vi "CameraSetting_AdvanceAttributesDisplay.vi"(8 "error in (no error)":errorcluster caption="错误输入（无错误）", 11 "当前可用相机":string(combo)) -> (0 "error out":errorcluster caption="错误输出")   [LabVIEW 2015]
panel:
  in  "主页按钮":bool
  in  "刷新按钮":bool
  out "相机属性参数列表":string[][](table)
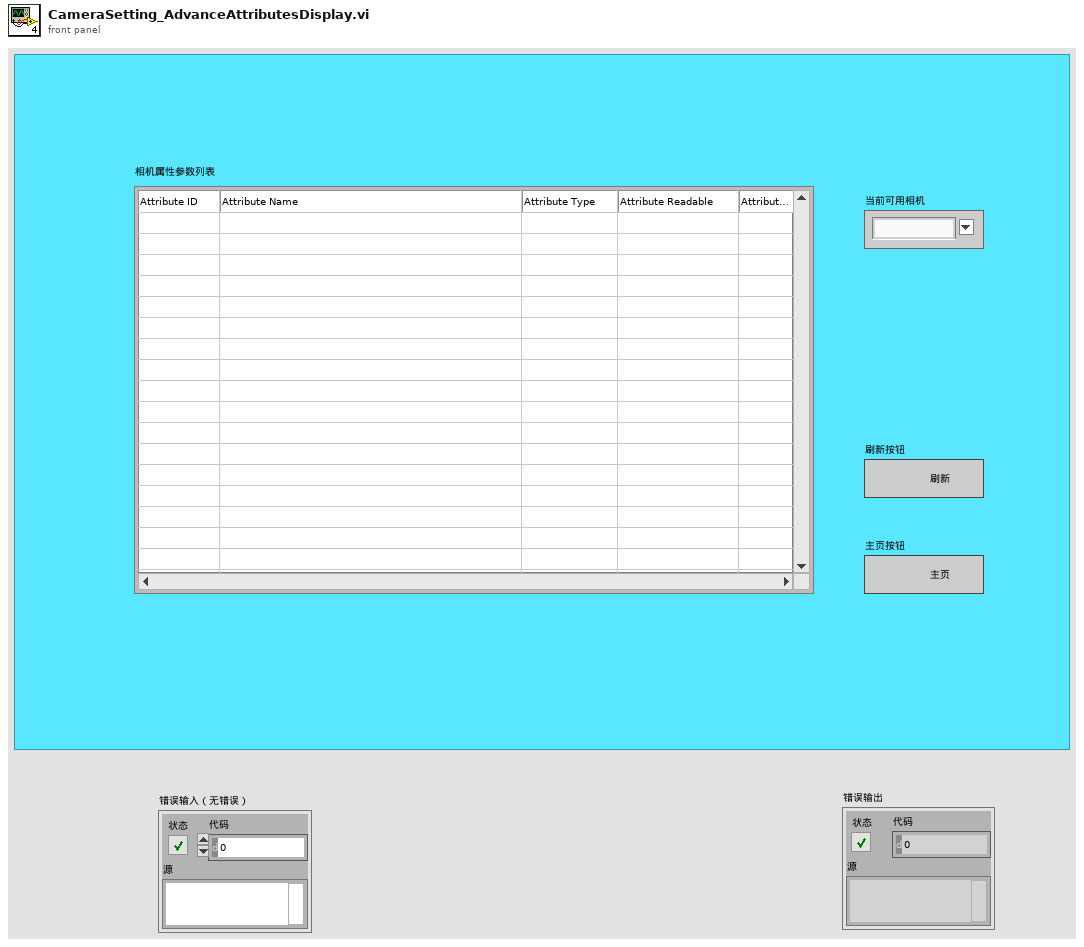
[diagram p1: front panel]
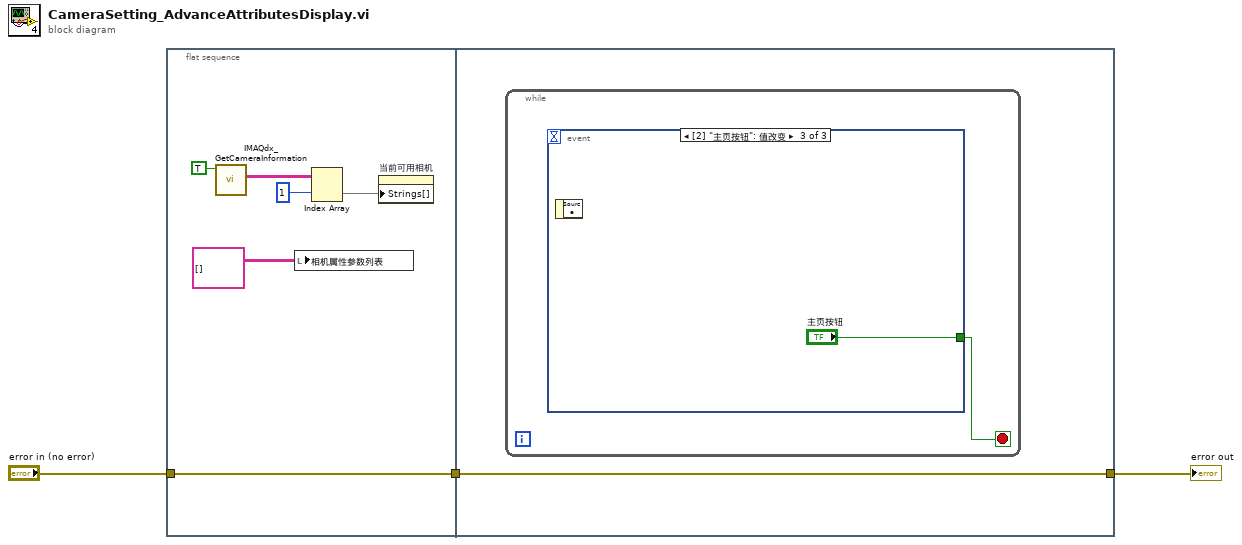
[diagram p0: block diagram]
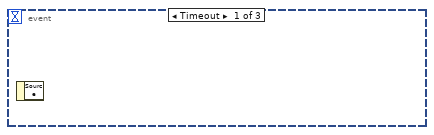
[diagram p2: hidden frame]
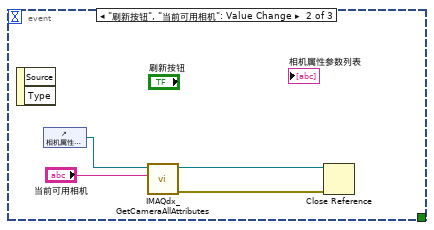
[diagram p3: hidden frame]
diagram:
  n1 = flat-sequence {
    tunnel: [w4] -> w3
    tunnel: "error in (no error)" -> [w4]
    tunnel: w3 -> [w10]
    tunnel: [w10] -> w1
    frame #0 {
      n2 = call "IMAQdx_GetCameraInformation.vi"("Connected Only? (Yes)"=TRUE) -> ("Camera Basic Information"=w9:string[][])  [unwired: 8 in, 2 out]
      n3 = local write "相机属性参数列表"(string[][] [] ("相机属性列表")) -> ()
      n4 = Index Array(array=w9, index (row)=1 ("索引 (行)")) -> (element=w7:string[])  [unwired: 1 in]
      n5 = property on="当前可用相机" class="CmbBox"("Strings[]"=w7) -> ()  [unwired: 2 in, 2 out]
    }
    frame #1 {
      n6 = while {
        stop <- w11 stop-if-true
        n7 = event shown="[2] \"主页按钮\": 值改变" {
          selector: _ -> [_ _ _]
          dyn-events: _ -> [_ _ _]
          timeout: _ -> [_ _ _]
          tunnel: [_ _ "主页按钮"] -> w11
          event Timeout {
            n8 = event-data() -> ()  [unwired: 1 in, 1 out]
          }
          event "刷新按钮", "当前可用相机": Value Change {
            n9 = event-data() -> ()  [unwired: 1 in, 2 out]
            n10 = control-ref of="相机属性参数列表"() -> (w14:refnum<vi>)
            n11 = call "IMAQdx_GetCameraAllAttributes.vi"("当前可用相机"="当前可用相机", "表格控件引用_输入"=w14) -> ("error out"=w12:errorcluster, "表格控件引用输出"=w13:refnum<vi>)  [unwired: 8 in]
            n12 = Close Reference(reference=w13, error in (no error)=w12) -> ()  [unwired: 1 out]
          }
          event "主页按钮": Value Change {
            n13 = event-data() -> ()  [unwired: 1 in, 1 out]
          }
        }
      }
    }
  }
  "error out" <- w1
